vi "Get Minimum Length.vi"(11 "Analog Waveform Array in":waveform(dbl)[](array[waveform])) -> (3 "Target Length":i32)   [LabVIEW 2018, in "Waveform Equalizer.lvlib"]
uses:
  Waveform Equalizer.lvlib
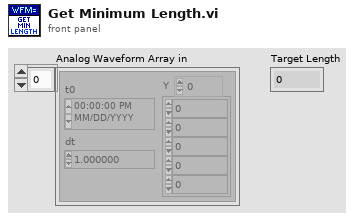
[diagram p1: front panel]
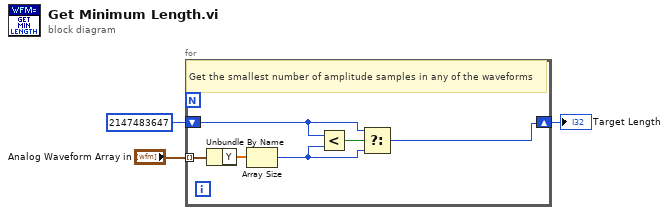
[diagram p0: block diagram]
diagram:
  n1 = for {
    tunnel: "Analog Waveform Array in" -> [w9] mode=indexing
    shift-right: [w5] -> w3
    shift-left: 2147483647 -> [w7]
    # "Get the smallest number of amplitude samples in any of the waveforms"
    n2 = Unbundle By Name(w9) -> ("Y"=w6:dbl[])
    n3 = Array Size(array=w6) -> (size(s)=w4:i32)
    n4 = Less?(x=w7, y=w4) -> (x < y?=w8:bool)
    n5 = Select(t=w7, s=w8, f=w4) -> (s? t:f=w5:i32)
  }
  "Target Length" <- w3
